vi "Revision Query.vi"(0 "VISA resource name":refnum<visa-resource-name>="COM1", 5 "Address (00)":i32 format="%0#2.0f", 11 "error in (no error)":errorcluster) -> (4 "VISA resource name out":refnum<visa-resource-name>, 6 "Pump status":T1 items=["Error - Can't read status"=-1, "Stopped"=0, "Infusing"=1, "Withdrawing"=2, "Pump stalled"=3, "Stopped at infuse limit"=4, "Stopped at withdraw limit"=5, "Emergency stop"=6, "Stopped at target volume"=7], 10 "Instrument Firmware Revision":string, 15 "error out":errorcluster)   [LabVIEW 2011]
doc: "This VI queries the current instrument firmware revision and instrument driver revision.\n\nModified from original which is Copyright 2005, National Instruments Corporation.\n\nModifications Copyright 2009, Jeff Gelles, Brandeis University"
uses:
  Pump status.ctl
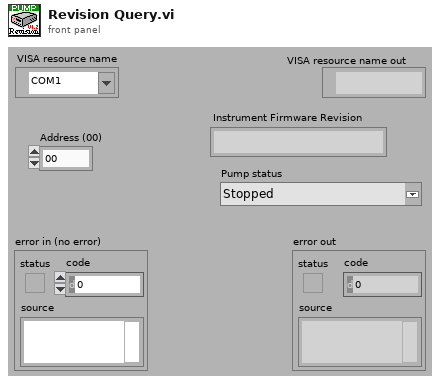
[diagram p1: front panel]
types:
  T1 = typedef "Pump status.ctl" = i8
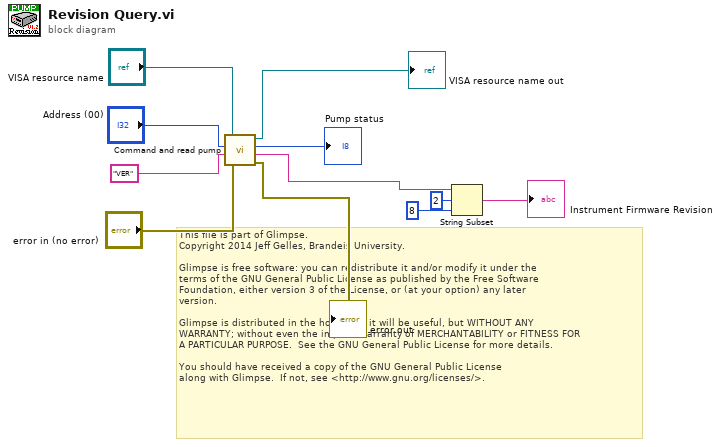
[diagram p0: block diagram]
diagram:
  # "This file is part of Glimpse. \nCopyright 2014 Jeff Gelles, Brandeis University.    \n\nGlimpse is free software: you can redistribute it and/or modify it under the \nterms of the GNU General Public License as published by the Free Software \nFoundation, either version 3 of the License, or (at your option) any later \nversion.\n\nGlimpse is distributed in the hope that it will be useful, but WITHOUT ANY \nWARRANTY; without even the implied warranty of MERCHANTABILITY or FITNESS FOR \nA PARTICULAR PURPOSE.  See the GNU General Public License for more details.\n\nYou should have received a copy of the GNU General Public License\nalong with Glimpse.  If not, see <http://www.gnu.org/licenses/>."
  n1 = call "Command and read pump.vi"("error in (no error)"="error in (no error)", "command"="VER" ("write buffer"), "Address (00)"="Address (00)", "VISA resource name"="VISA resource name") -> ("error out"=→"error out":errorcluster, "Output String"=w2:string, "Pump status"=→"Pump status":T1, "VISA resource name out"=→"VISA resource name out":refnum<visa-resource-name>)
  n2 = String Subset(string=w2, offset (0)=2, length (rest)=8 ("length (rest)")) -> (substring=→"Instrument Firmware Revision":string)
